vi "read_Variable.vi"(2 "error in (no error)":errorcluster, 3 "Variable Cluster":T1) -> (0 "error out":errorcluster, 1 "dup Variable Cluster":T1)   [LabVIEW 2012, in "HGF_SV.lvlib" / "HGF_SVMonitor.lvclass"]
doc: "This VI reads a shared variable by Datasocket. Shared variable must be a string including the prefix (opc:, psp:, ds:). The Datasocket_read Vi is configured to read with no time out and not waiting for updated value."
uses:
  HGF_SVMonitor.lvclass
  HGF_BaseClasses/HGF_NetworkVisitor/HGF_NetworkVisitor.lvclass
  HGF_BaseClasses/HGF_TriggeredEvent/HGF_TriggeredEvent.lvclass
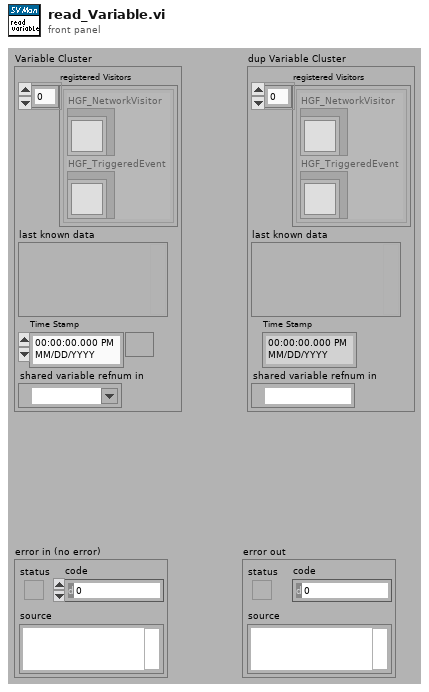
[diagram p1: front panel]
types:
  T1 = cluster{"registered Visitors":cluster{"HGF_NetworkVisitor":refnum<class "HGF_NetworkVisitor.lvclass">, "HGF_TriggeredEvent":refnum<class "HGF_TriggeredEvent.lvclass">}[], "last known data":variant, "Time Stamp":timestamp, "shared variable refnum in":refnum<k21>}
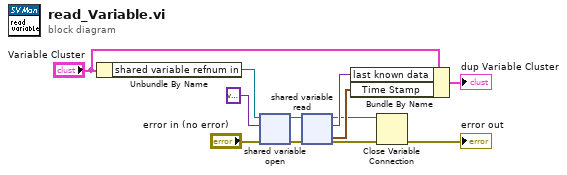
[diagram p0: block diagram]
diagram:
  n1 = Unbundle By Name("Variable Cluster") -> ("shared variable refnum in"=w7:refnum<k21>)
  n2 = shared-variable-open(w7, "error in (no error)", variant ("variant")) -> (w6:refnum<k21>, w4:errorcluster)  [unwired: 1 in]
  n3 = shared-variable-read(w6, w4) -> (w3:refnum<k21>, w2:errorcluster, w11:variant, w10:timestamp)
  n4 = Bundle By Name(cluster="Variable Cluster", "last known data"=w11, "Time Stamp"=w10) -> (→"dup Variable Cluster":T1)
  n5 = Close Variable Connection(8:w2, 11:w3) -> (0:→"error out":errorcluster)
